vi "Global Value.vi"() -> ()   [LabVIEW 2018]
panel:
  out "접속":bool
  out "CommConnect":i32
  out "다우존스":string[](array[string])
  out "나스닥":string[](array[string])
  out "S&P500":string[](array[string])
  out "니케이":string[](array[string])
  out "코스피":string[](array[string])
  out "가격급등락":string[][](array[string])
  out "고저가근접":string[][](array[string])
  out "상하한가":string[][](array[string])
  out "신고저가":string[][](array[string])
  out "종목수(자동)":string
  out "보유주식(자동)":string[][](array[string])
  out "Data 5":string[][](array[string])
  out "Data 14":string[][](array[string])
  out "Data 13":string[][](array[string])
  out "Data 12":string[][](array[string])
  out "Data 11":string[][](array[string])
  out "Data 10":string[][](array[string])
  out "Data 9":string[][](array[string])
  out "Data 8":string[][](array[string])
  out "Data 7":string[][](array[string])
  out "Data 6":string[][](array[string])
  out "10 호가":string[](array[string])
  out "이벤트 데이터 2":T1
  out "주문":string[](array[string])
  out "보유주식":string[][](array[string])
  out "잔고":string[](array[string])
  out "Data 4":string[][](array[string])
  out "Data 3":string[][](array[string])
  out "Data 2":string[][](array[string])
  out "Data 1":string[][](array[string])
  out "Data":string[][](array[string])
  in  "접속 문자열":string
  # "접속"
  # "주요지수"
  # "관심주"
  # "30일 Data 분석"
  # "특징주"
  # "10호가"
  # "잔고"
  # "주문"
  # "자동매매"
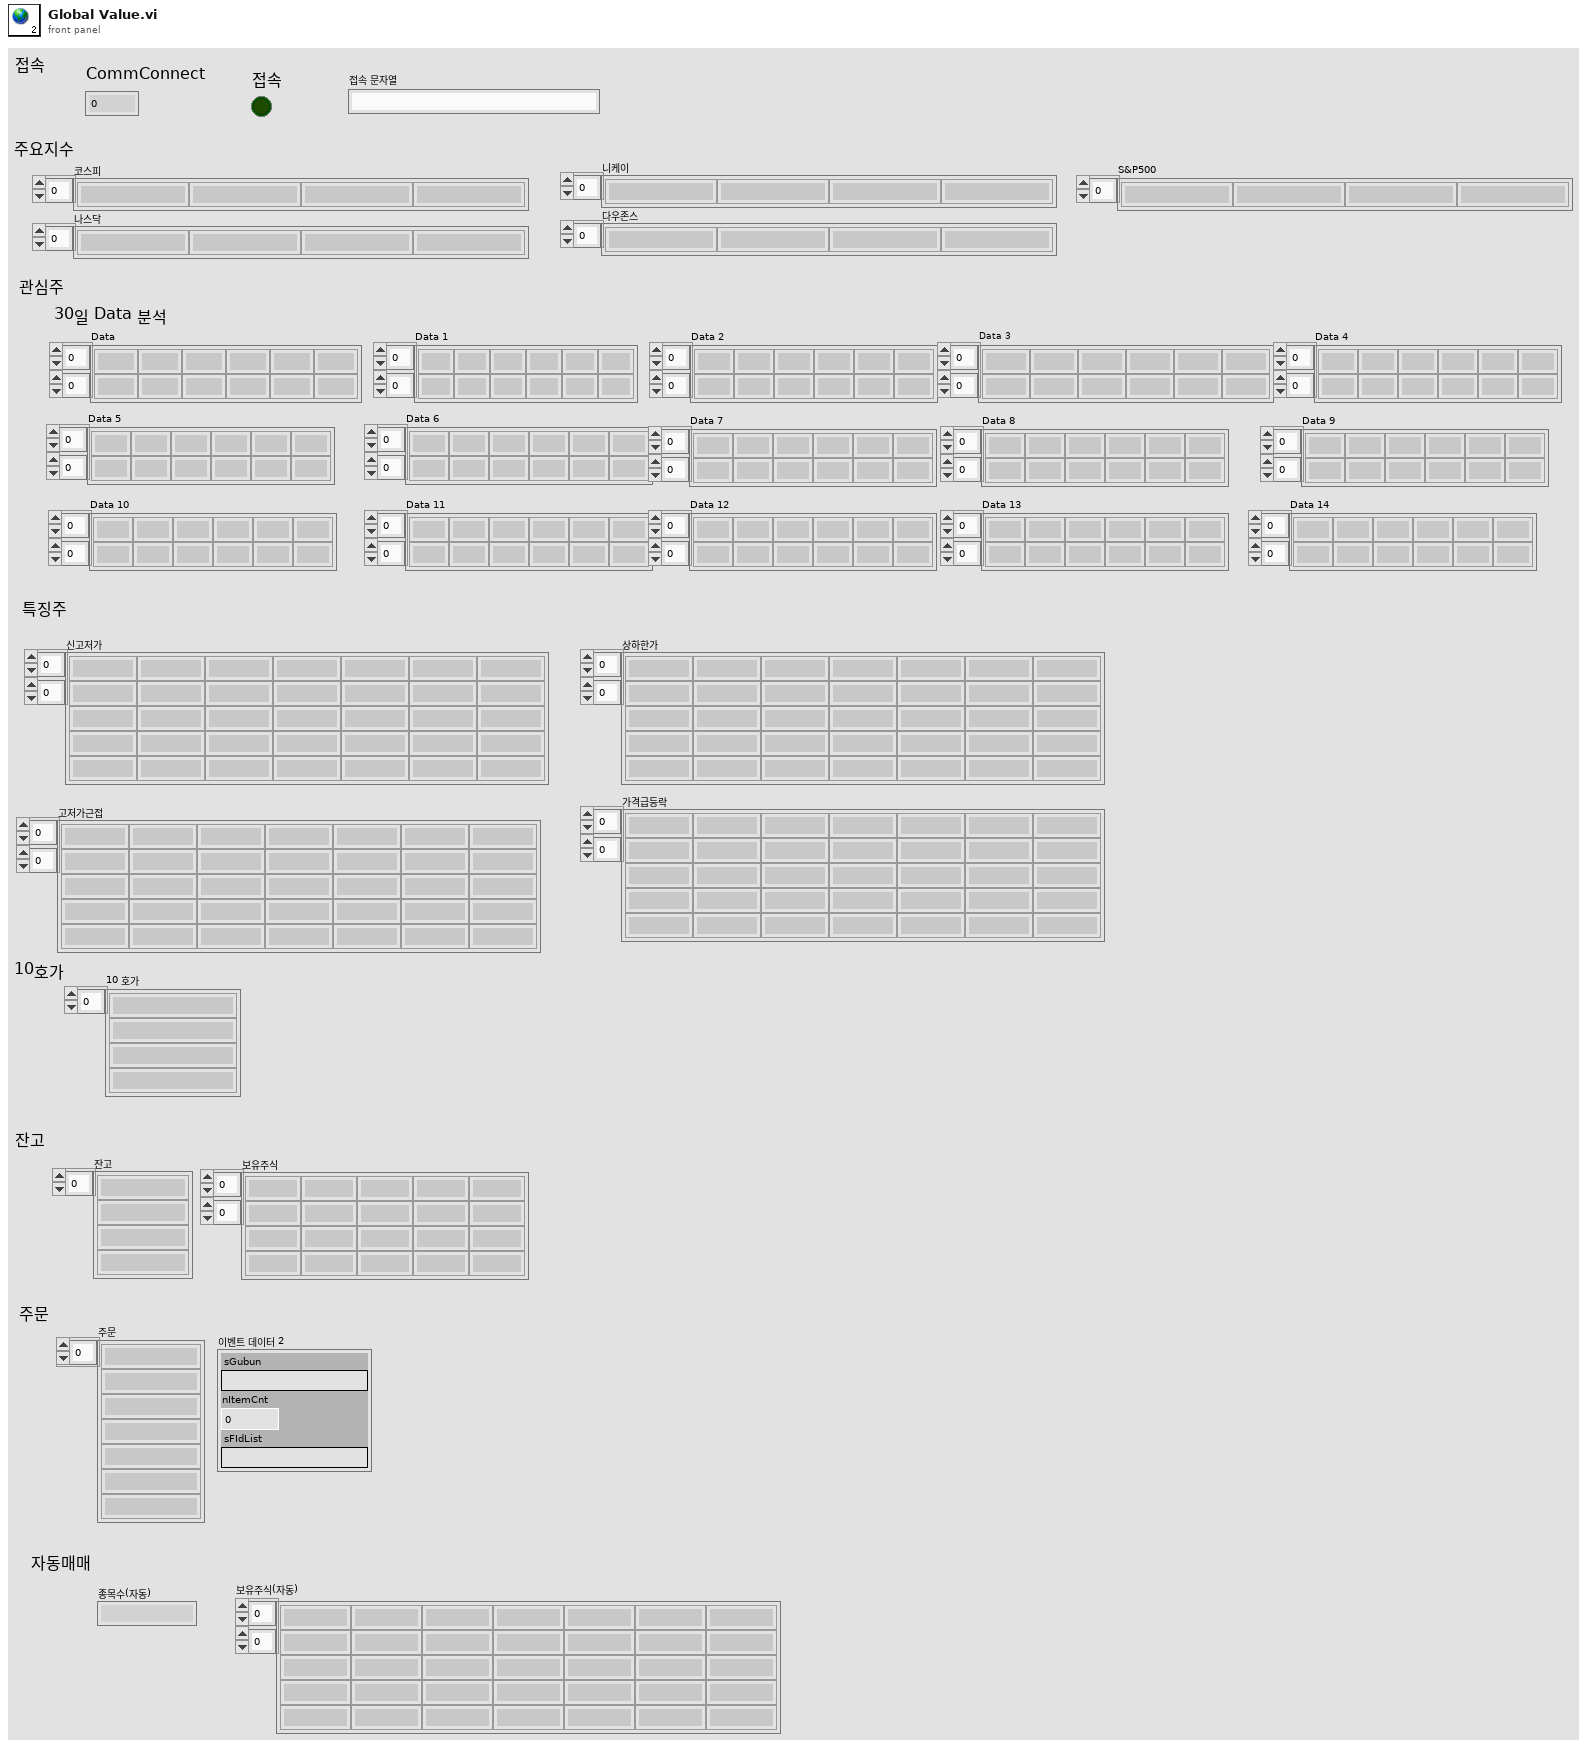
[diagram p1: front panel]
types:
  T1 = cluster{"sGubun":string, "nItemCnt":i32, "sFIdList":string}
diagram:
